vi "Init.vi"(8 "error in (no error)":errorcluster, 10 "Index":i32, 11 "Group":refnum<class "Group BOOL.lvclass">) -> (0 "error out":errorcluster, 3 "Channel BOOL out":refnum<class "Channel BOOL.lvclass">)   [LabVIEW 2020, in "Vecto.lvlib" / "Channel BOOL.lvclass"]
uses:
  Channel BOOL.lvclass
  Channel BOOL.lvclass/Channel BOOL.ctl
  Group BOOL/Group BOOL.lvclass
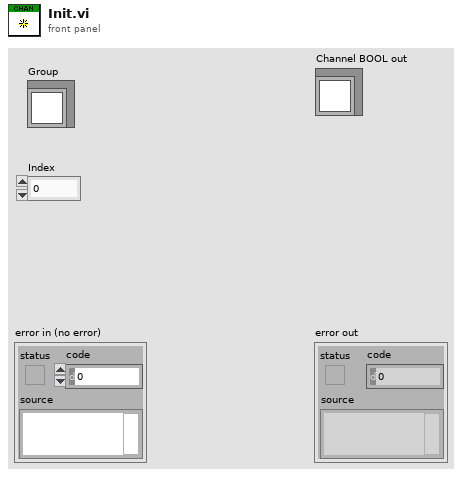
[diagram p1: front panel]
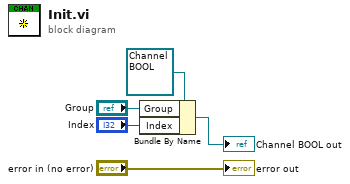
[diagram p0: block diagram]
diagram:
  n1 = Bundle By Name(cluster=refnum<class "Channel BOOL.lvclass"> refnum ("Channel BOOL in"), "Group"="Group", "Index"="Index") -> (→"Channel BOOL out":refnum<class "Channel BOOL.lvclass">)
  "error out" <- "error in (no error)"
